vi "Pre Launch Init.vi"(11 "Nested Actor in":refnum<class "Nested Actor.lvclass">) -> (0 "error out":errorcluster, 3 "Nested Actor out":refnum<class "Nested Actor.lvclass">)   [LabVIEW 2020, in "Nested Actor.lvlib" / "Nested Actor.lvclass"]
doc: "(<B>Filename</B>: Actor Framework.lvlib:Actor.lvclass:Pre Launch Init.vi)\n\nDefines behavior that occurs after the Launch Nested Actor method is invoked but before the actor's Actor Core method begins running.\n\nBy default, this method does nothing. A descendant class may override it to define behavior."
uses:
  Nested Actor.lvclass
  Nested Actor.lvclass/Nested Actor.ctl
  <vilib>/ActorFramework/Actor/Actor.lvclass
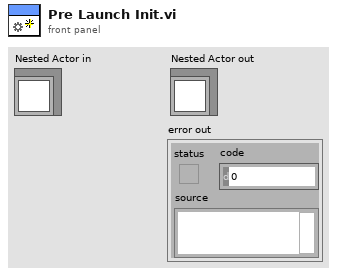
[diagram p1: front panel]
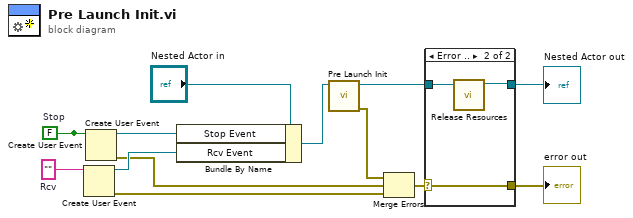
[diagram p0: block diagram]
diagram:
  w13 = ""  # Rcv
  w8 = FALSE  # Stop
  n1 = Create User Event(user event datatype=w13) -> (user event=w11:refnum<user-event>, error out=w9:errorcluster)  [unwired: 1 in]
  n2 = Create User Event(user event datatype=w8) -> (user event=w12:refnum<user-event>, error out=w10:errorcluster)  [unwired: 1 in]
  n3 = Create User Event(user event datatype=w8) -> ()  [unwired: 1 in, 2 out]
  n4 = Bundle By Name(cluster="Nested Actor in", "Stop Event"=w12, "Rcv Event"=w11) -> (w6:refnum<class "Nested Actor.lvclass">)
  n5 = call-parent "Pre Launch Init.vi"("Actor in"=w6) -> ("error out"=w5:errorcluster, "Actor out"=w2:refnum<class "Nested Actor.lvclass">)  [unwired: 9 in]
  n6 = Merge Errors(w5, w10, w9) -> (w4:errorcluster)
  n7 = case shown="Error .." w4 {
    selector: w4 -> [w15 w18]
    tunnel: [w15 w18] -> w3
    tunnel: w2 -> [w14 w17]
    tunnel: [w14 w16] -> w1
    frame No Error {
    }
    frame Error {
      n8 = call "Release Resources.vi"("Nested Actor in"=w17) -> ("Nested Actor out"=w16:refnum<class "Nested Actor.lvclass">)  [unwired: 10 in]
    }
  }
  "error out" <- w3
  "Nested Actor out" <- w1
